vi "ThemalImaging(VDAQ)2.vi"() -> ()   [LabVIEW 2011]
uses:
  <vilib>/vision/Image Controls.llb/IMAQ Image.ctl
  <vilib>/Analysis/1siggen.llb/Riffle Array (I32).vi
  <vilib>/Analysis/NI_AALBase.lvlib
  <vilib>/vision/NI_Vision_Development_Module.lvlib
panel:
  out "数值":i32
  out "OnlineMap Array":T1[](array[typedef])
  out "Hue":i32
  out "Saturation":i32
  out "DR/R array":T1[](array[typedef])
  out "停止循环":bool
  out "imaging通知器输出":refnum<notifier>
  out "DeInitDSPs":i32
  out "错误输出":errorcluster
  in  "Stimuli":i32=5
  in  "FrameHeight":i32=576
  in  "FrameWidth":i32=704
  in  "选项卡控件":enum32{"前面板", "参数设置", "OnLineMap", "mask"}(tab)
  out "log":string
  out "Image":T1(plugin-control)
  out "Stim_ID":i32(listbox)=1
  in  "开始/暂停":bool=TRUE
  in  "停止":bool
  out "重排的 Stim ID":i32[](array[numeric]) caption="重排的{X}"
  out "重排的 Stim ID Index":i32[](array[numeric]) caption="重排的索引"
  in  "Contrast":i32(slide) min=0 max=127 scale=0.0..127.0
  in  "Brightness":i32(slide) min=0 max=255 scale=0.0..255.0
  in  "上限温度":dbl=32.5
  in  "下限温度":dbl=20.6
  out "当前点温度":dbl
  out "Histogram Graph":T2(graph) caption="直方图"
  out "校正循环计时":dbl caption="已用时间(s)"
  out "校准":bool
  out "start calibrate":bool
  out "wait calibrate":bool
  out "block":i32
  in  "FramesPerStim(25Hz)":i32=100
  in  "Blk目录":path=path "D:/_expt/111110_C27/Run_02_G4_ThemalImaging"
  in  "文件名":string="G4_E05"
  in  "TimeForPrepare(ms)":u32=1000
  in  "stim ID":u8[](array[numeric])=[0, 2, 4, 6, 8]
  in  "blk总数":i32=500
  in  "stim protocol":T3(array[ring])=[enum."prep stim", enum."wait calibrate", enum."wait respirator", enum."show stim", enum."recording data", enum."Blank stim", enum."write data", enum."DR/R", enum."ISI"]
  in  "blank stim":u8
  in  "wait（ms）":u32=10
  in  "ISI（ms）":u32=8000
  in  "stim 循环时间/秒":dbl=10.0
  in  "OnlineMap":cluster{"数组 1":i32[], "数组 2":i32[]}[](array[cluster])=[{"数组 1"=[2], "数组 2"=[6]}, {"数组 1"=[4], "数组 2"=[8]}, {"数组 1"=[2, 6], "数组 2"=[4, 8]}, {"数组 1"=[2, 4, 6, 8], "数组 2"=[0]}, {"数组 1"=[2, 4], "数组 2"=[6, 8]}]
  in  "DR/R parameter":T4={"frame_zero_0"=0, "frame_zero_1"=10, "frame_0"=40, "frame_1"=80}
  in  "mask 1":T1(plugin-control)=refnum
  in  "mask 2":T1(plugin-control)=refnum
  # "运行60秒后再开始"
  # "÷"
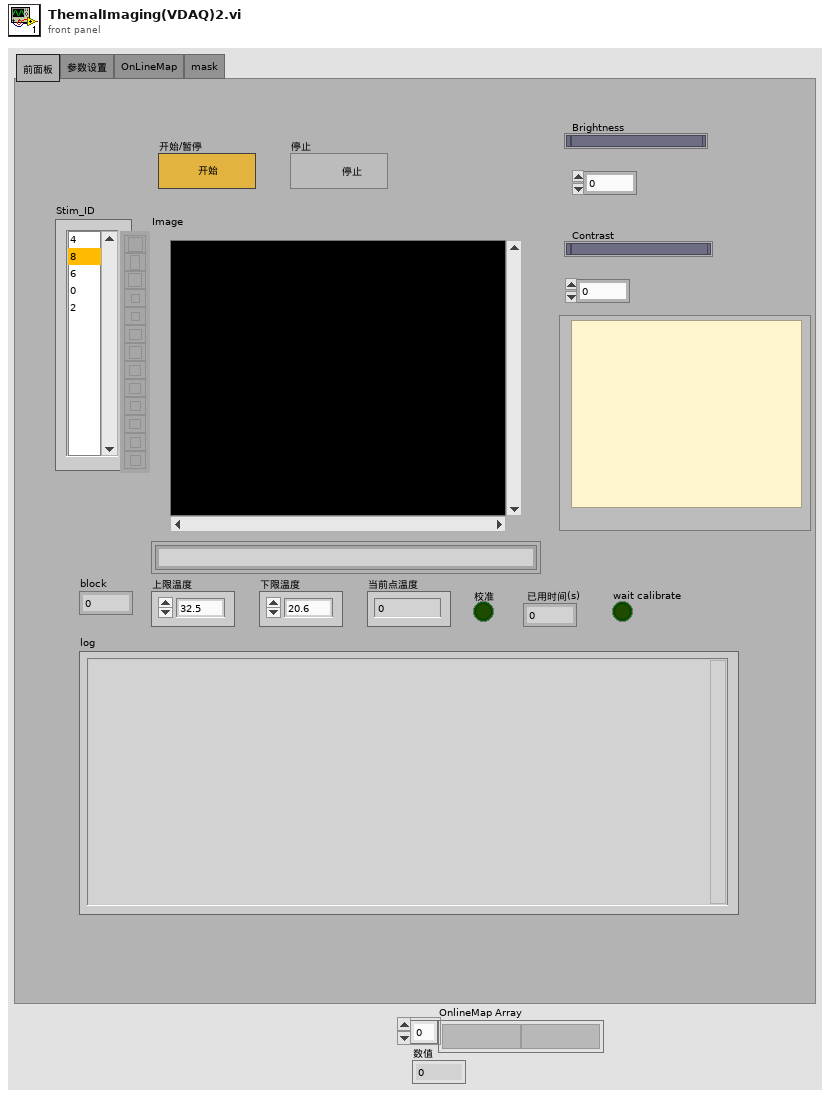
[diagram p1: front panel]
types:
  T1 = typedef "IMAQ Image.ctl" = refnum<image>
  T2 = cluster{"X Values":dbl[], "Histogram: h(x)":i32[]}
  T3 = enum16{"wait", "prep stim", "show stim", "wait respirator", "recording data", "write data", "Blank stim", "wait heart", "ISI", "DR/R", "wait calibrate"}[]
  T4 = cluster{"frame_zero_0":i32, "frame_zero_1":i32, "frame_0":i32, "frame_1":i32}
  T5 = typedef "Image Type" = u32
  T6 = enum16{"big-endian, network order", "native, host order", "little-endian"}
  T7 = cluster{"Mean Value":sgl, "Standard Variation":sgl, "Minimal Value":sgl, "Maximal Value":sgl, "Area (calibrated)":sgl, "Area (pixels)":u32, "%":sgl, "Calibration Valid":bool}
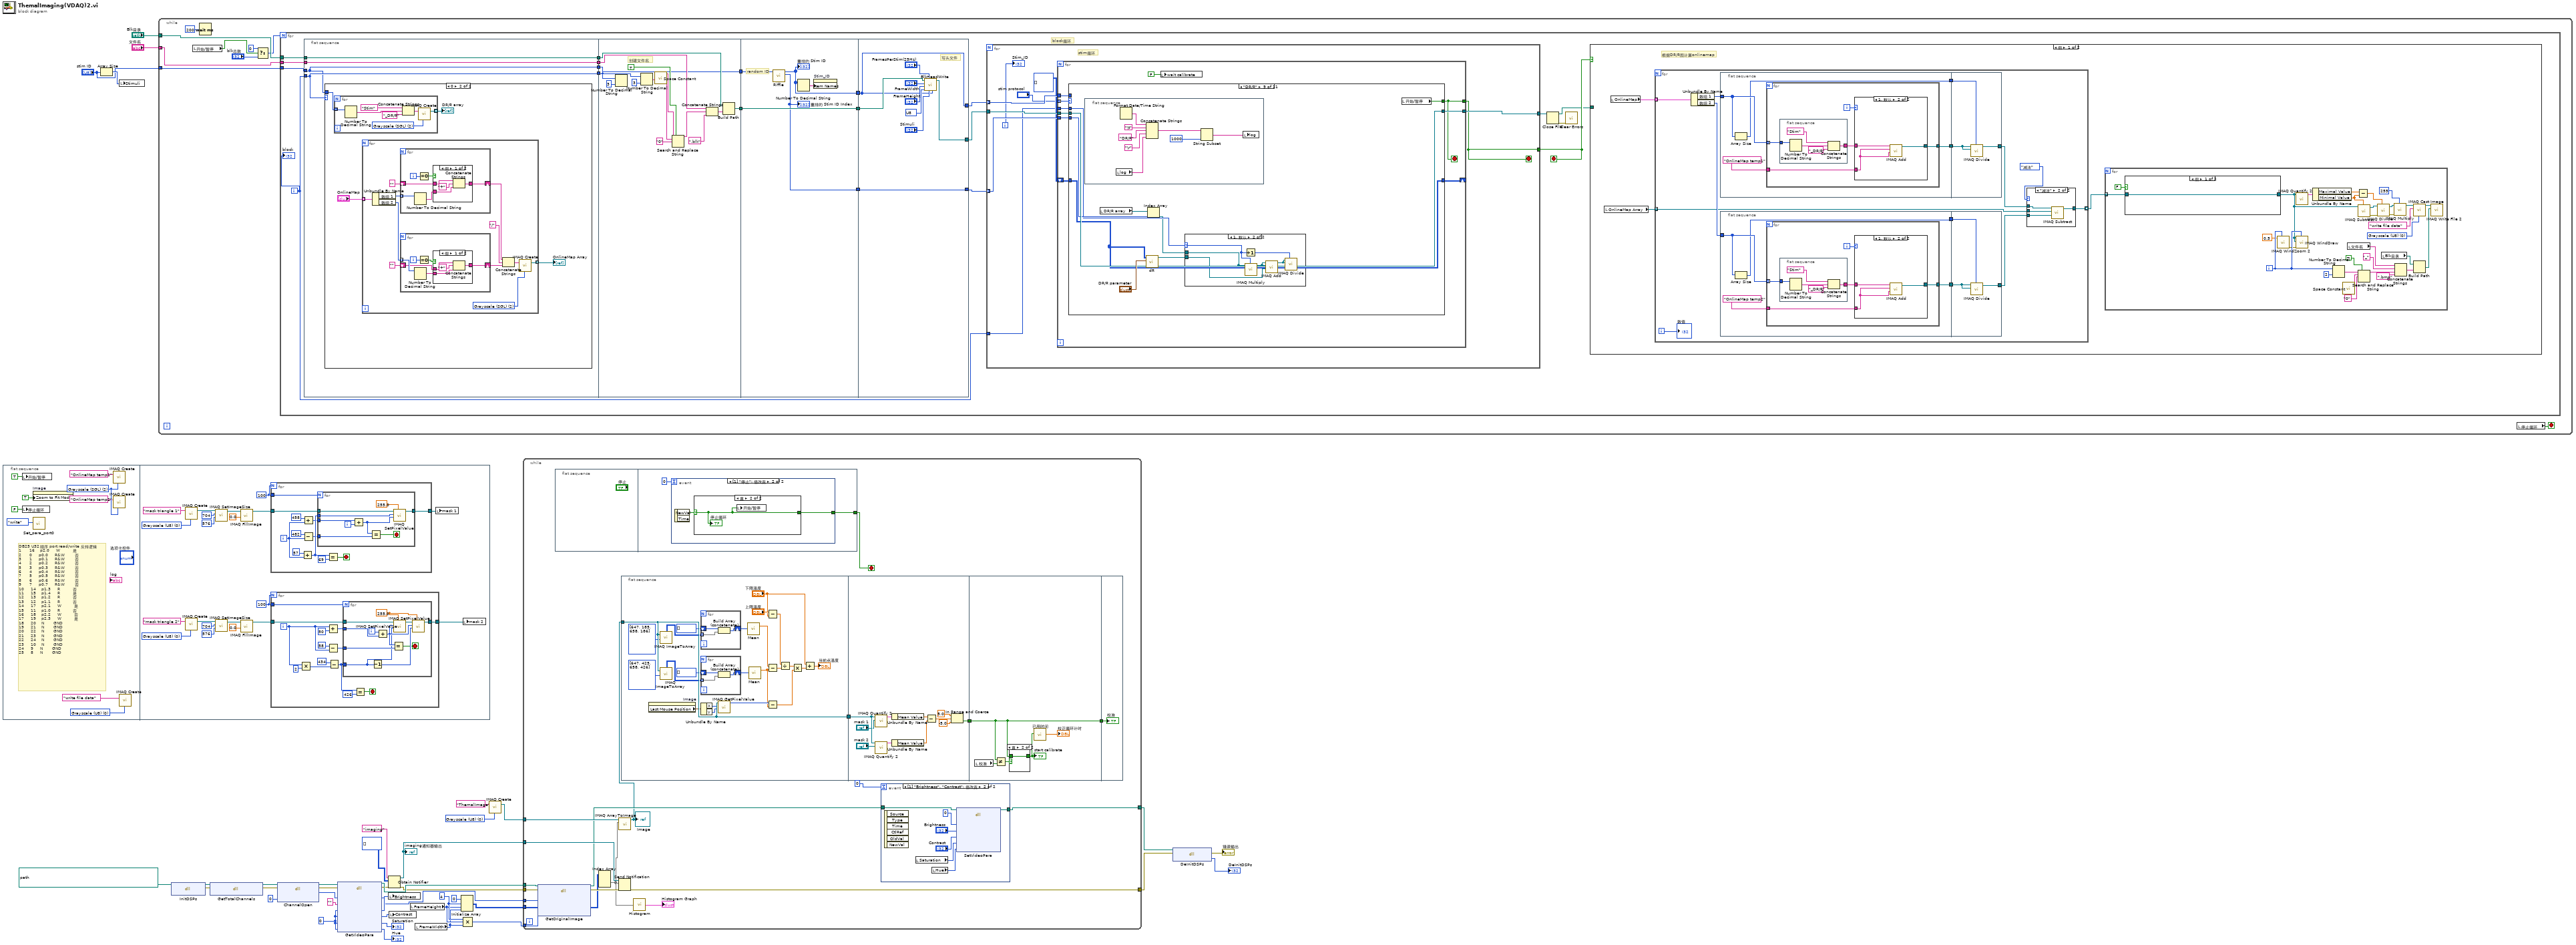
[diagram p0: block diagram]
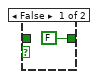
[diagram p2: hidden frame]
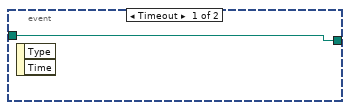
[diagram p3: hidden frame]
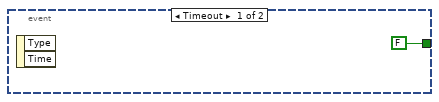
[diagram p4: hidden frame]
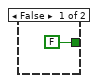
[diagram p5: hidden frame]
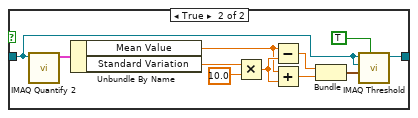
[diagram p6: hidden frame]
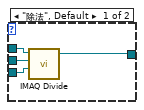
[diagram p7: hidden frame]
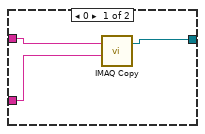
[diagram p8: hidden frame]
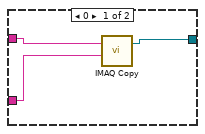
[diagram p9: hidden frame]
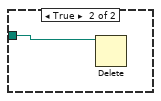
[diagram p10: hidden frame]
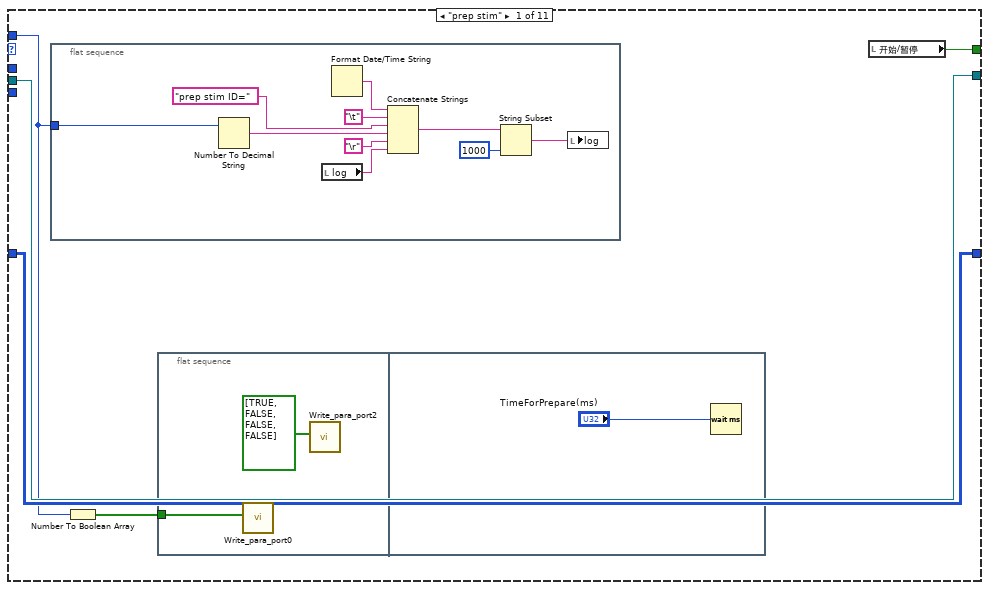
[diagram p14: hidden frame]
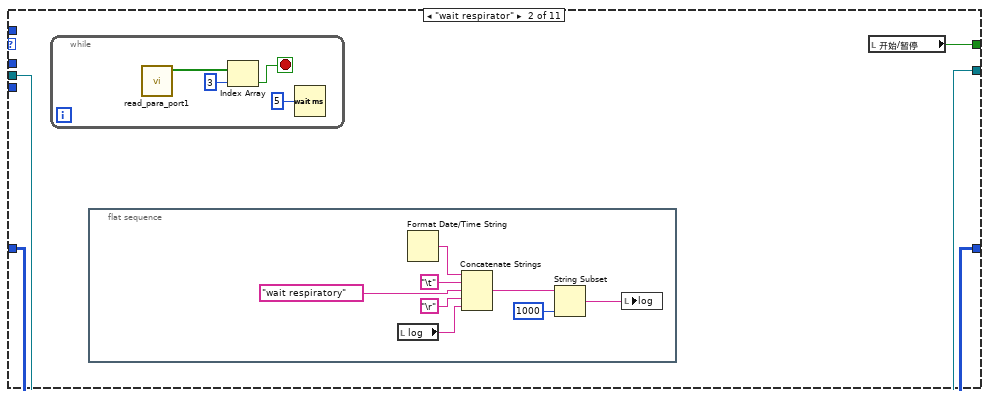
[diagram p15: hidden frame]
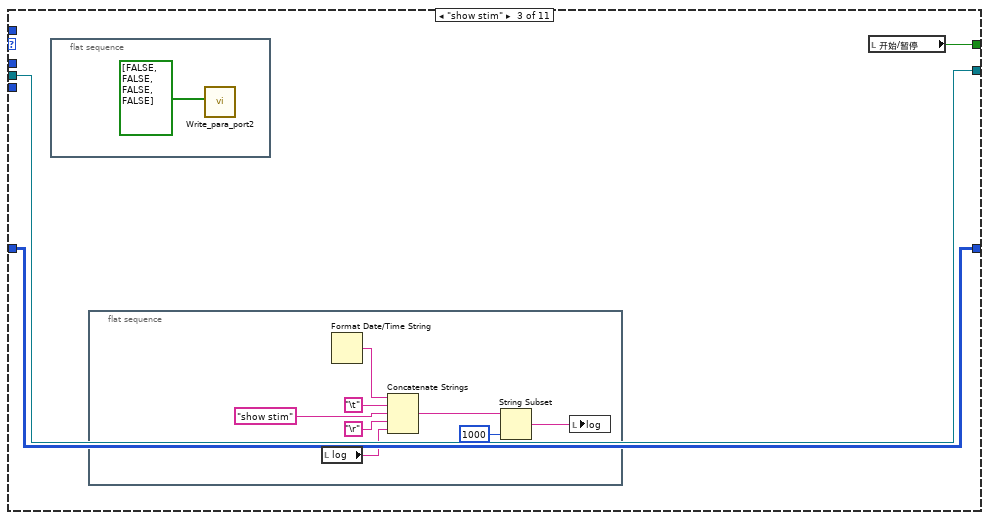
[diagram p16: hidden frame]
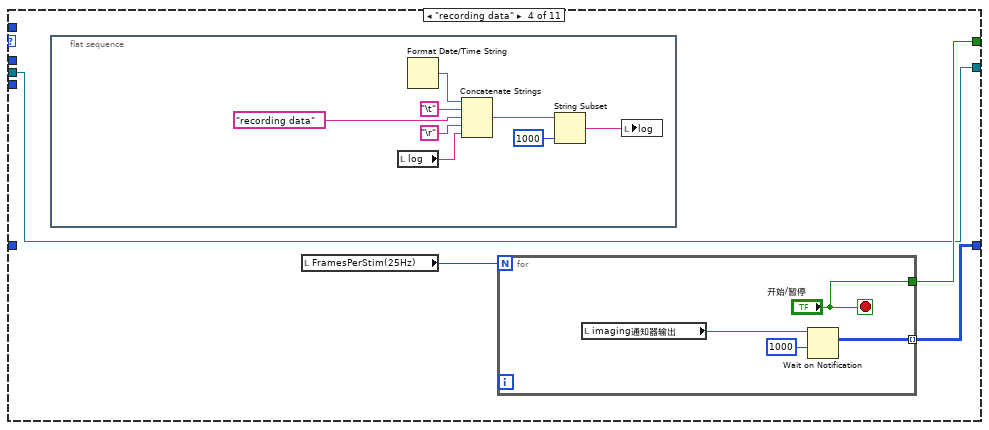
[diagram p17: hidden frame]
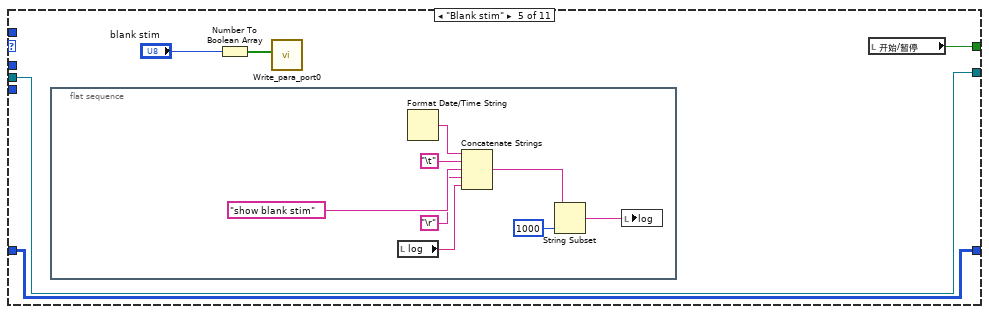
[diagram p18: hidden frame]
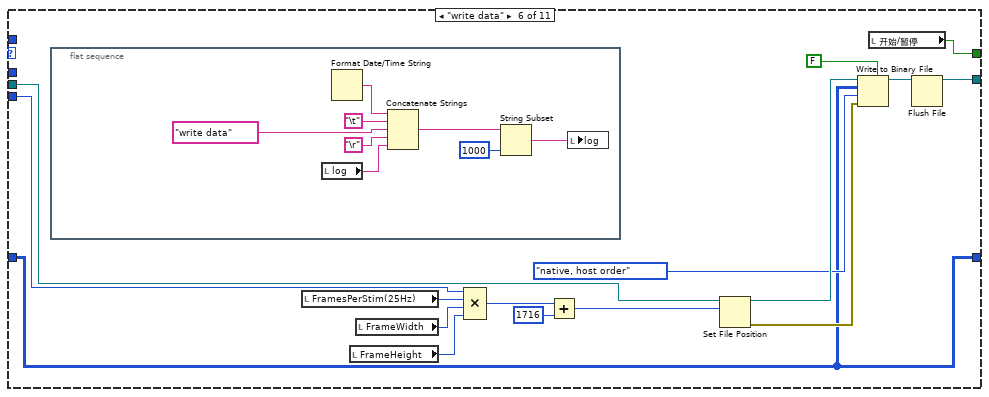
[diagram p19: hidden frame]
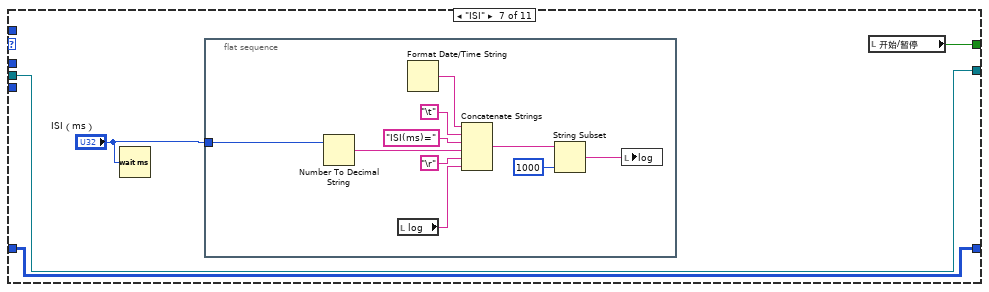
[diagram p20: hidden frame]
diagram:
  w17 = 4 ("元素")
  w34 = T5 0 items=["Grayscale (U8)", "Grayscale (I16)", "Grayscale (SGL)", "Complex (CSG)", "RGB (U32)", "HSL (U32)", "RGB (U64)", "Grayscale (U16)"] ("Image Type")
  w23 = 0 ("Brightness")
  n1 = flat-sequence {
    frame #0 {
      w40 = T5 0 items=["Grayscale (U8)", "Grayscale (I16)", "Grayscale (SGL)", "Complex (CSG)", "RGB (U32)", "HSL (U32)", "RGB (U64)", "Grayscale (U16)"] ("Image Type")
      w43 = T5 2 items=["Grayscale (U8)", "Grayscale (I16)", "Grayscale (SGL)", "Complex (CSG)", "RGB (U32)", "HSL (U32)", "RGB (U64)", "Grayscale (U16)"] ("Image Type")
      # "DB25\tU32顺序\tport\tread/write\t反转逻辑\n1\t     16\t   p2.0    \tW\t        是\n2\t     0    \tp0.0\t   \tR&W\t      否\n3\t     1\t\t   p0.1\t   \tR&W      \t否\n4\t\t    2\t   \tp0.2   \t\tR&W      \t否\n5\t\t    3\t\t   p0.3   \t\tR&W\t      否\n6\t\t    4\t   \tp0.4   \t\tR&W      \t否\n7\t\t    5\t   \tp0.5   \t\tR&W      \t否\n8\t\t    6\t   \tp0.6\t   \tR&W      \t否\n9\t    \t7\t   \tp0.7\t   \tR&W\t      否\n10\t    14   \tp1.3   \t\tR        \t否\n11\t   \t15   \tp1.4   \t\tR        \t是\n12\t   \t13   \tp1.2\t   \tR        \t否\n13    \t12   \tp1.1\t   \tR        \t否\n14     17   \tp2.1\t   \tW        \t是\n15    \t11   \tp1.0   \t\tR\t        否\n16    \t18   \tp2.2   \t\tW        \t否\n17    \t19\t   p2.3   \t\tW\t        是\n18    \t20   \tN   \t  \tGND\t\n19    \t21   \tN   \t  \tGND\t\n20\t    22\t   N\t  \t  \tGND\t\n21\t    23\t   N  \t  \t\tGND\t\n22\t    24\t   N  \t  \t\tGND\t\n23    \t10   \tN  \t  \t\tGND\t\n24    \t9\t    N  \t  \t\tGND\t\n25\t    8    \tN  \t  \t\tGND"
      n2 = local write "开始/暂停"(TRUE ("开始/暂停")) -> ()
      n3 = local write "停止循环"(FALSE ("开始/暂停")) -> ()
      n4 = property on="Image" class="ImageControl"("Zoom to Fit Mode"=TRUE) -> ()  [unwired: 2 in, 2 out]
      n5 = call "Set_para_port0.vi"("R or W"=enum16{"read", "write"}."write") -> ()  [unwired: 9 in, 2 out]
      n6 = call "IMAQ Create"("Image Name"="OnlineMap temp1", "Image Type"=w43) -> ()  [unwired: 3 in, 2 out]
      n7 = call "IMAQ Create"("Image Name"="OnlineMap temp2", "Image Type"=w43) -> ()  [unwired: 3 in, 2 out]
      n8 = call "IMAQ Create"("Image Name"="write file data", "Image Type"=w40) -> ()  [unwired: 3 in, 2 out]
    }
    frame #1 {
      w50 = 100
      w57 = T5 0 items=["Grayscale (U8)", "Grayscale (I16)", "Grayscale (SGL)", "Complex (CSG)", "RGB (U32)", "HSL (U32)", "RGB (U64)", "Grayscale (U16)"] ("Image Type")
      w60 = 100
      w67 = T5 0 items=["Grayscale (U8)", "Grayscale (I16)", "Grayscale (SGL)", "Complex (CSG)", "RGB (U32)", "HSL (U32)", "RGB (U64)", "Grayscale (U16)"] ("Image Type")
      n9 = call "IMAQ Create"("Image Name"="mask triangle 1", "Image Type"=w67) -> ("New Image"=w66:T1)  [unwired: 3 in, 1 out]
      n10 = call "IMAQ Create"("Image Name"="mask triangle 2", "Image Type"=w57) -> ("New Image"=w56:T1)  [unwired: 3 in, 1 out]
      n11 = call "IMAQ SetImageSize"("Y Resolution"=576, "X Resolution"=704, "Image"=w66) -> ("Image Out"=w63:T1)  [unwired: 2 in, 1 out]
      n12 = call "IMAQ SetImageSize"("Y Resolution"=576, "X Resolution"=704, "Image"=w56) -> ("Image Out"=w53:T1)  [unwired: 2 in, 1 out]
      n13 = call "IMAQ FillImage"("Pixel Value (U8, U16, I16, Float)"=sgl 0.0, "Image"=w63) -> ("Image Out"=w61:T1)  [unwired: 8 in, 1 out]
      n14 = call "IMAQ FillImage"("Pixel Value (U8, U16, I16, Float)"=sgl 0.0, "Image"=w53) -> ("Image Out"=w51:T1)  [unwired: 8 in, 1 out]
      n15 = for {
        N: w60 -> [_]
        tunnel: w60 -> [w105]
        tunnel: [w104] -> w59
        tunnel: w61 -> [w103]
        i -> [w95]
        stop <- w99 stop-if-true
        n16 = Add(x=57 ("X Coordinate"), y=w95) -> (x+y=w101:i32)
        n17 = Add(x=458 ("Y Coordinate"), y=w95) -> (x+y=w97:i32)
        n18 = Subtract(x=482 ("y"), y=w95) -> (x-y=w94:i32)
        n19 = for {
          N: w105 -> [_]
          tunnel: w103 -> [w114]
          tunnel: [w112] -> w104
          tunnel: w101 -> [w108]
          tunnel: w97 -> [w107]
          tunnel: w94 -> [w106]
          i -> [w111]
          stop <- w109 stop-if-true
          n20 = Add(x=w107, y=w111) -> (x+y=w110:i32)
          n21 = Equal?(x=w110, y=w106) -> (x = y?=w109:bool)
          n22 = call "IMAQ SetPixelValue"("Pixel Value"=sgl 255.0, "Y Coordinate"=w110, "X Coordinate"=w108, "Image"=w114) -> ("Image Out"=w112:T1)  [unwired: 6 in, 1 out]
        }
        n23 = Equal?(x=w101, y=69) -> (x = y?=w99:bool)
      }
      n24 = for {
        N: w50 -> [_]
        tunnel: w50 -> [w82]
        tunnel: [w81] -> w49
        tunnel: w51 -> [w80]
        i -> [w74]
        stop <- w69 stop-if-true
        n25 = Multiply(x=w74, y=2) -> (x*y=w72:i32)
        n26 = Add(x=w74, y=50 ("X Coordinate")) -> (x+y=w78:i32)
        n27 = Subtract(x=58 ("y"), y=w74) -> (x-y=w76:i32)
        n28 = Subtract(x=434 ("Y Coordinate"), y=w72) -> (x-y=w71:i32)
        n29 = for {
          N: w82 -> [_]
          tunnel: w80 -> [w93]
          tunnel: [w90] -> w81
          tunnel: w78 -> [w86]
          tunnel: w76 -> [w85]
          tunnel: w71 -> [w84]
          i -> [w92]
          stop <- w87 stop-if-true
          w83 = sgl 255.0 ("Pixel Value")
          n30 = Decrement(x=w84) -> (x-1=w89:i32)
          n31 = Add(x=w92, y=w86) -> (x+y=w88:i32)
          n32 = Equal?(x=w88, y=w85) -> (x = y?=w87:bool)
          n33 = call "IMAQ SetPixelValue"("Pixel Value"=w83, "Y Coordinate"=w84, "X Coordinate"=w88, "Image"=w93) -> ("Image Out"=w91:T1)  [unwired: 6 in, 1 out]
          n34 = call "IMAQ SetPixelValue"("Pixel Value"=w83, "Y Coordinate"=w89, "X Coordinate"=w88, "Image"=w91) -> ("Image Out"=w90:T1)  [unwired: 6 in, 1 out]
        }
        n35 = Equal?(x=w71, y=426) -> (x = y?=w69:bool)
      }
      n36 = local write "mask 1"(w59) -> ()
      n37 = local write "mask 2"(w49) -> ()
    }
  }
  n38 = Array Size(array="stim ID") -> (size(s)=w37:i32)
  n39 = local write "Stimuli"(w37) -> ()
  n40 = while {
    tunnel: "stim ID" -> [w123]
    tunnel: "文件名" -> [w122]
    tunnel: "Blk目录" -> [w121]
    stop <- w119 stop-if-true
    n41 = local read "开始/暂停"() -> (w118:bool)
    n42 = Wait (ms)(milliseconds to wait=u32 200 ("等待时间（毫秒）")) -> ()  [unwired: 1 out]
    n43 = Select(t=0, s=w118, f="blk总数") -> (s? t:f=w115:i32)
    n44 = for {
      N: w115 -> [_]
      tunnel: w123 -> [w128]
      tunnel: w122 -> [w143]
      tunnel: w121 -> [w142]
      i -> [w132]
      stop <- w134 stop-if-true
      # "block循环"
      n45 = flat-sequence {
        tunnel: w142 -> [w260]
        tunnel: w143 -> [w261]
        tunnel: w132 -> [w259]
        tunnel: [w259] -> w131
        tunnel: [w261] -> w130
        tunnel: [w260] -> w129
        tunnel: w128 -> [w258]
        tunnel: [w258] -> w126
        tunnel: [w307] -> w140
        tunnel: w131 -> [w313]
        tunnel: w130 -> [w312]
        tunnel: w129 -> [w308]
        tunnel: [w306] -> w127
        tunnel: w126 -> [w306]
        tunnel: w140 -> [w324]
        tunnel: [w324] -> w139
        tunnel: [w322] -> w138
        tunnel: w127 -> [w321]
        tunnel: [w320] -> w125
        tunnel: w139 -> [w328]
        tunnel: [w327] -> w141
        tunnel: w138 -> [w326]
        tunnel: [w326] -> w137
        tunnel: w125 -> [w325]
        tunnel: [w325] -> w124
        frame #0 {
          n46 = case shown="0" w259 {
            tunnel: w258 -> [_ w265]
            frame 1, Default {
            }
            frame 0 {
              n47 = for {
                tunnel: w265 -> [w302] mode=indexing
                tunnel: [w299] -> w264 mode=indexing
                w305 = T5 2 items=["Grayscale (U8)", "Grayscale (I16)", "Grayscale (SGL)", "Complex (CSG)", "RGB (U32)", "HSL (U32)", "RGB (U64)", "Grayscale (U16)"] ("Image Type")
                n48 = Number To Decimal String(number=w302) -> (decimal integer string=w303:string)  [unwired: 1 in]
                n49 = Concatenate Strings("Stim", w303, "_DR/R" ("字符串")) -> (w300:string)
                n50 = call "IMAQ Create"("Image Name"=w300, "Image Type"=w305) -> ("New Image"=w299:T1)  [unwired: 3 in, 1 out]
              }
              "DR/R array" <- w264
              n51 = for {
                tunnel: "OnlineMap" -> [w276] mode=indexing
                tunnel: [w266] -> w262 mode=indexing
                w274 = T5 2 items=["Grayscale (U8)", "Grayscale (I16)", "Grayscale (SGL)", "Complex (CSG)", "RGB (U32)", "HSL (U32)", "RGB (U64)", "Grayscale (U16)"] ("Image Type")
                n52 = Unbundle By Name(w276) -> ("数组 1"=w275:i32[], "数组 2"=w271:i32[])
                n53 = for {
                  tunnel: w275 -> [w291] mode=indexing
                  shift-right: [w289] -> w272
                  shift-left: "" -> [w288]
                  i -> [w293]
                  n54 = Number To Decimal String(number=w291) -> (decimal integer string=w290:string)  [unwired: 1 in]
                  n55 = Equal To 0?(x=w293) -> (x = 0?=w292:bool)
                  n56 = case shown="假" w292 {
                    tunnel: w290 -> [w294 w298]
                    tunnel: [w297 w298] -> w289
                    tunnel: w288 -> [w296 _]
                    frame False {
                      n57 = Concatenate Strings(w296, "+" ("字符串"), w294) -> (w297:string)
                    }
                    frame True {
                    }
                  }
                }
                n58 = for {
                  tunnel: w271 -> [w280] mode=indexing
                  shift-right: [w278] -> w269
                  shift-left: "" -> [w277]
                  i -> [w282]
                  n59 = Number To Decimal String(number=w280) -> (decimal integer string=w279:string)  [unwired: 1 in]
                  n60 = Equal To 0?(x=w282) -> (x = 0?=w281:bool)
                  n61 = case shown="假" w281 {
                    tunnel: w279 -> [w283 w287]
                    tunnel: [w286 w287] -> w278
                    tunnel: w277 -> [w285 _]
                    frame False {
                      n62 = Concatenate Strings(w285, "+" ("字符串"), w283) -> (w286:string)
                    }
                    frame True {
                    }
                  }
                }
                n63 = Concatenate Strings(w272, "/" ("字符串"), w269) -> (w267:string)
                n64 = call "IMAQ Create"("Image Name"=w267, "Image Type"=w274) -> ("New Image"=w266:T1)  [unwired: 3 in, 1 out]
              }
              "OnlineMap Array" <- w262
            }
          }
        }
        frame #1 {
          # "创建文件名"
          n65 = Number To Decimal String(number=w313, width (-)=i16 3 ("宽度(-)")) -> ()  [unwired: 1 out]
          n66 = Number To Decimal String(number=w313, width (-)=i16 3 ("宽度(-)")) -> (decimal integer string=w315:string)
          n67 = call <vilib>:"Space Constant.vi"() -> ("String"=w316:string)
          n68 = Search and Replace String(replace all?=TRUE ("替换全部？(F)"), input string=w315, search string=w316, replace string="0" ("替换字符串(\"\")")) -> (result string=w311:string)  [unwired: 4 in, 3 out]
          n69 = Concatenate Strings(w312, w311, ".blk" ("字符串")) -> (w309:string)
          n70 = Build Path(base path=w308, name or relative path=w309) -> (appended path=w307:path)
        }
        frame #2 {
          # "random ID"
          n71 = call-poly <vilib>:"Riffle.vi"("X"=w321) -> ("Riffled Index"=w320:i32[], "Riffled {X}"=w322:i32[])  [unwired: 8 in, 1 out]
          "重排的 Stim ID Index" <- w320
          "重排的 Stim ID" <- w322
          n72 = Number To Decimal String(number=w322) -> (decimal integer string=w323:string[])  [unwired: 1 in]
          n73 = property on="Stim_ID" class="LstBox (严格)"("Item Names"=w323) -> ()  [unwired: 2 in, 2 out]
        }
        frame #3 {
          w331 = u16 11 items=["U8"=11, "I16"=12, "U32"=13, "SGL"=14] ("datatype")
          # "写头文件"
          n74 = call "BlkHeadWrite.vi"("SequenceOfID"=w326, "Stimuli"="Stimuli", "FramesPerStim"="FramesPerStim(25Hz)", "datatype"=w331, "FrameHeight"="FrameHeight", "FrameWidth"="FrameWidth", "BlkFilePath"=w328) -> ("引用句柄输出"=w327:refnum<file>)  [unwired: 4 in]
        }
      }
      n75 = for {
        tunnel: w141 -> [w342]
        tunnel: [w340] -> w135
        tunnel: w124 -> [w341] mode=indexing
        tunnel: w137 -> [w339] mode=indexing
        tunnel: [w338] -> w134
        tunnel: w132 -> [w334]
        i -> [w337]
        stop <- w338 stop-if-true
        # "stim循环"
        n76 = for {
          tunnel: w341 -> [w351]
          tunnel: w339 -> [w349]
          tunnel: [w345] -> w338
          shift-right: [w348] -> _
          shift-left: u8[][][] [] ("初始化的数组") -> [w347]
          tunnel: "stim protocol" -> [w346] mode=indexing
          tunnel: w342 -> [w352]
          tunnel: [w350] -> w340
          tunnel: w334 -> [w344]
          stop <- w345 stop-if-true
          n77 = case shown="\"DR/R\"" w346 {
            tunnel: w352 -> [w354 w371 w386 w398 w414 w442 w452 w466 w486 w504 w522]
            tunnel: w351 -> [_ _ _ _ _ w441 _ _ w484 _ _]
            tunnel: [w354 w371 w386 w398 w414 w429 w452 w466 w486 w504 w522] -> w350
            tunnel: w349 -> [w353 _ _ _ _ _ _ _ _ _ _]
            tunnel: [w355 w372 w387 w400 w415 w427 w453 w467 w485 w505 w515] -> w345
            tunnel: [w356 w373 w388 w399 w416 w428 w454 w468 w479 w506 w521] -> w348
            tunnel: w347 -> [w356 w373 w388 _ w416 w428 w454 w468 w479 w506 w521]
            tunnel: w344 -> [_ _ _ _ _ _ _ _ w483 _ _]
            frame "prep stim" {
              n78 = flat-sequence {
                tunnel: w353 -> [w365]
                frame #0 {
                  n79 = Number To Decimal String(number=w365) -> (decimal integer string=w364:string)  [unwired: 1 in]
                  n80 = local read "log"() -> (w360:string)
                  n81 = Format Date/Time String() -> (date/time string=w367:string)  [unwired: 3 in]
                  n82 = Concatenate Strings(w367, "\t", "prep stim ID=" ("字符串"), w364, "\r", w360) -> (w362:string)
                  n83 = String Subset(string=w362, length (rest)=1000 ("y")) -> (substring=w361:string)  [unwired: 1 in]
                  n84 = local write "log"(w361) -> ()
                }
              }
              n85 = Number To Boolean Array(number=w353) -> (Boolean array=w357:bool[])
              n86 = flat-sequence {
                tunnel: w357 -> [w369]
                frame #0 {
                  n87 = call "Write_para_port0.vi"("port0（8元素）"=w369) -> ()  [unwired: 10 in, 1 out]
                  n88 = call "Write_para_port2.vi"("port2（4元素）"=bool[] [TRUE, FALSE, FALSE, FALSE] ("port2")) -> ()  [unwired: 10 in, 1 out]
                }
                frame #1 {
                  n89 = Wait (ms)(milliseconds to wait="TimeForPrepare(ms)") -> ()  [unwired: 1 out]
                }
              }
              n90 = local read "开始/暂停"() -> (w355:bool)
            }
            frame "wait respirator" {
              n91 = while {
                stop <- w383 stop-if-true
                n92 = call "read_para_port1.vi"() -> ("port1（5元素）"=w385:bool[])  [unwired: 10 in, 1 out]
                n93 = Index Array(array=w385, index=3 ("索引")) -> (element=w383:bool)
                n94 = Wait (ms)(milliseconds to wait=u32 5 ("等待时间（毫秒）")) -> ()  [unwired: 1 out]
              }
              n95 = flat-sequence {
                frame #0 {
                  n96 = local read "log"() -> (w376:string)
                  n97 = Format Date/Time String() -> (date/time string=w381:string)  [unwired: 3 in]
                  n98 = Concatenate Strings(w381, "\t", "wait respiratory" ("字符串"), "\r", w376) -> (w378:string)
                  n99 = String Subset(string=w378, length (rest)=1000 ("y")) -> (substring=w377:string)  [unwired: 1 in]
                  n100 = local write "log"(w377) -> ()
                }
              }
              n101 = local read "开始/暂停"() -> (w372:bool)
            }
            frame "show stim" {
              n102 = flat-sequence {
                frame #0 {
                  n103 = call "Write_para_port2.vi"("port2（4元素）"=bool[] [FALSE, FALSE, FALSE, FALSE] ("port2")) -> ()  [unwired: 10 in, 1 out]
                }
              }
              n104 = flat-sequence {
                frame #0 {
                  n105 = local read "log"() -> (w391:string)
                  n106 = Format Date/Time String() -> (date/time string=w396:string)  [unwired: 3 in]
                  n107 = Concatenate Strings(w396, "\t", "show stim" ("字符串"), "\r", w391) -> (w393:string)
                  n108 = String Subset(string=w393, length (rest)=1000 ("y")) -> (substring=w392:string)  [unwired: 1 in]
                  n109 = local write "log"(w392) -> ()
                }
              }
              n110 = local read "开始/暂停"() -> (w387:bool)
            }
            frame "recording data" {
              n111 = flat-sequence {
                frame #0 {
                  n112 = local read "log"() -> (w404:string)
                  n113 = Format Date/Time String() -> (date/time string=w409:string)  [unwired: 3 in]
                  n114 = Concatenate Strings(w409, "\t", "recording data" ("字符串"), "\r", w404) -> (w406:string)
                  n115 = String Subset(string=w406, length (rest)=1000 ("y")) -> (substring=w405:string)  [unwired: 1 in]
                  n116 = local write "log"(w405) -> ()
                }
              }
              n117 = local read "FramesPerStim(25Hz)"() -> (w401:i32)
              n118 = for {
                N: w401 -> [_]
                tunnel: [w412] -> w399 mode=indexing
                tunnel: ["开始/暂停"] -> w400
                stop <- "开始/暂停" stop-if-true
                n119 = local read "imaging通知器输出"() -> (w413:refnum<notifier>)
                n120 = Wait on Notification(notifier=w413, timeout in ms (-1)=1000 ("超时毫秒(-1)")) -> (notification=w412:u8[][])  [unwired: 2 in, 3 out]
              }
            }
            frame "Blank stim" {
              n121 = flat-sequence {
                frame #0 {
                  n122 = local read "log"() -> (w421:string)
                  n123 = Format Date/Time String() -> (date/time string=w426:string)  [unwired: 3 in]
                  n124 = Concatenate Strings(w426, "\t", "show blank stim" ("字符串"), "\r", w421) -> (w423:string)
                  n125 = String Subset(string=w423, length (rest)=1000 ("y")) -> (substring=w422:string)  [unwired: 1 in]
                  n126 = local write "log"(w422) -> ()
                }
              }
              n127 = Number To Boolean Array(number="blank stim") -> (Boolean array=w417:bool[])
              n128 = call "Write_para_port0.vi"("port0（8元素）"=w417) -> ()  [unwired: 10 in, 1 out]
              n129 = local read "开始/暂停"() -> (w415:bool)
            }
            frame "write data" {
              n130 = flat-sequence {
                frame #0 {
                  n131 = local read "log"() -> (w445:string)
                  n132 = Format Date/Time String() -> (date/time string=w450:string)  [unwired: 3 in]
                  n133 = Concatenate Strings(w450, "\t", "write data" ("字符串"), "\r", w445) -> (w447:string)
                  n134 = String Subset(string=w447, length (rest)=1000 ("y")) -> (substring=w446:string)  [unwired: 1 in]
                  n135 = local write "log"(w446) -> ()
                }
              }
              n136 = local read "FramesPerStim(25Hz)"() -> (w433:i32)
              n137 = local read "FrameHeight"() -> (w431:i32)
              n138 = local read "FrameWidth"() -> (w432:i32)
              n139 = Compound Arithmetic op=MULTIPLY(w441, w433, w432, w431) -> (w436:i32)
              n140 = Add(x=w436, y=i64 1716 ("偏移量（字节）（0）")) -> (x+y=w434:i64)
              n141 = Set File Position(offset (in bytes) (0)=w434, refnum=w442) -> (refnum out=w439:refnum<file>, error out=w437:errorcluster)  [unwired: 2 in]
              n142 = Write to Binary File(file (use dialog)=w439, data=w428, error in=w437, 5:FALSE ("预置数组或字符串大小？(T)"), 9:T6."native, host order" ("字节顺序(0:big-endian, network order)")) -> (refnum out=w430:refnum<file>)  [unwired: 1 in, 2 out]
              n143 = local read "开始/暂停"() -> (w427:bool)
              n144 = Flush File(refnum=w430) -> (refnum out=w429:refnum<file>)  [unwired: 1 in, 1 out]
            }
            frame "ISI" {
              n145 = Wait (ms)(milliseconds to wait="ISI（ms）") -> ()  [unwired: 1 out]
              n146 = flat-sequence {
                tunnel: "ISI（ms）" -> [w458]
                frame #0 {
                  n147 = Number To Decimal String(number=w458) -> (decimal integer string=w462:string)  [unwired: 1 in]
                  n148 = local read "log"() -> (w457:string)
                  n149 = Format Date/Time String() -> (date/time string=w464:string)  [unwired: 3 in]
                  n150 = Concatenate Strings(w464, "\t", "ISI(ms)=" ("字符串"), w462, "\r", w457) -> (w460:string)
                  n151 = String Subset(string=w460, length (rest)=1000 ("y")) -> (substring=w459:string)  [unwired: 1 in]
                  n152 = local write "log"(w459) -> ()
                }
              }
              n153 = local read "开始/暂停"() -> (w453:bool)
            }
            frame "wait", Default {
              n154 = Wait (ms)(milliseconds to wait="wait（ms）") -> ()  [unwired: 1 out]
              n155 = flat-sequence {
                tunnel: "wait（ms）" -> [w472]
                frame #0 {
                  n156 = Number To Decimal String(number=w472) -> (decimal integer string=w476:string)  [unwired: 1 in]
                  n157 = local read "log"() -> (w471:string)
                  n158 = Format Date/Time String() -> (date/time string=w478:string)  [unwired: 3 in]
                  n159 = Concatenate Strings(w478, "\t", "wait(ms)=" ("字符串"), w476, "\r", w471) -> (w474:string)
                  n160 = String Subset(string=w474, length (rest)=1000 ("y")) -> (substring=w473:string)  [unwired: 1 in]
                  n161 = local write "log"(w473) -> ()
                }
              }
              n162 = local read "开始/暂停"() -> (w467:bool)
            }
            frame "DR/R" {
              n163 = flat-sequence {
                frame #0 {
                  n164 = local read "log"() -> (w490:string)
                  n165 = Format Date/Time String() -> (date/time string=w495:string)  [unwired: 3 in]
                  n166 = Concatenate Strings(w495, "\t", "DR/R" ("字符串"), "\r", w490) -> (w492:string)
                  n167 = String Subset(string=w492, length (rest)=1000 ("y")) -> (substring=w491:string)  [unwired: 1 in]
                  n168 = local write "log"(w491) -> ()
                }
              }
              n169 = local read "DR/R array"() -> (w480:T1[])
              n170 = call "dR.vi"("DR/R parameter"="DR/R parameter", "数组"=w479) -> ("Image Dst Out"=w482:T1)  [unwired: 9 in]
              n171 = Index Array(array=w480, index=w484) -> (element=w481:T1)
              n172 = case shown="1, 默认" w483 {
                selector: w483 -> [_ w500]
                tunnel: w482 -> [w497 w501]
                tunnel: w481 -> [w496 w503]
                frame 0 {
                  n173 = call "IMAQ Copy"("Image Dst"=w496, "Image Src"=w497) -> ()  [unwired: 4 in, 2 out]
                }
                frame 1, Default {
                  n174 = Increment(x=w500) -> (x+1=w499:i32)
                  n175 = call "IMAQ Multiply"("Image Src A"=w503, "Constant"=w500, "Image Dst"=w503) -> ("Image Dst Out"=w502:T1)  [unwired: 4 in, 1 out]
                  n176 = call "IMAQ Add"("Image Src A"=w502, "Image Dst"=w502, "Image Src B"=w501) -> ("Image Dst Out"=w498:T1)  [unwired: 4 in, 1 out]
                  n177 = call "IMAQ Divide"("Image Src A"=w498, "Constant"=w499, "Image Dst"=w498) -> ()  [unwired: 4 in, 2 out]
                }
              }
              n178 = local read "开始/暂停"() -> (w485:bool)
            }
            frame "wait heart" {
              n179 = flat-sequence {
                frame #0 {
                  n180 = local read "log"() -> (w509:string)
                  n181 = Format Date/Time String() -> (date/time string=w514:string)  [unwired: 3 in]
                  n182 = Concatenate Strings(w514, "\t", "wait heart" ("字符串"), "\r", w509) -> (w511:string)
                  n183 = String Subset(string=w511, length (rest)=1000 ("y")) -> (substring=w510:string)  [unwired: 1 in]
                  n184 = local write "log"(w510) -> ()
                }
              }
              n185 = local read "开始/暂停"() -> (w505:bool)
            }
            frame "wait calibrate" {
              n186 = local read "校正循环计时"() -> (w520:dbl)
              n187 = Subtract(x=60.0, y=w520) -> (x-y=w518:dbl)
              n188 = Less Or Equal?(x=w518, y="stim 循环时间/秒") -> (x <= y?=w516:bool)
              n189 = case shown="真" w516 {
                selector: w516 -> [_ w525]
                tunnel: [FALSE ("开始/暂停") w524] -> w515
                frame False {
                }
                frame True {
                  n190 = flat-sequence {
                    tunnel: [w526] -> w524
                    frame #0 {
                      n191 = while {
                        tunnel: [w527] -> w526
                        stop <- w528 stop-if-true
                        n192 = local read "start calibrate"() -> (w529:bool)
                        n193 = local read "开始/暂停"() -> (w527:bool)
                        n194 = Wait (ms)(milliseconds to wait=u32 5 ("等待时间（毫秒）")) -> ()  [unwired: 1 out]
                        n195 = Or(x=w529, y=w527) -> (x .or. y?=w528:bool)
                      }
                    }
                    frame #1 {
                      n196 = Wait (ms)(milliseconds to wait=u32 3000 ("等待时间（毫秒）")) -> ()  [unwired: 1 out]
                    }
                  }
                  "wait calibrate" <- w525
                }
              }
            }
          }
          n197 = local write "wait calibrate"(FALSE ("wait calibrate")) -> ()
        }
        "Stim_ID" <- w337
      }
      n198 = Close File(refnum=w135) -> (path=w133:path, error out=w136:errorcluster)  [unwired: 1 in]
      n199 = call <vilib>:"Clear Errors.vi"("error in (no error)"=w136) -> ()  [unwired: 6 in, 1 out]
      n200 = case shown="假" w134 {
        tunnel: w133 -> [_ w257]
        frame False {
          # "根据DR/R图计算onlinemap"
          n201 = local read "OnlineMap Array"() -> (w145:T1[])
          n202 = local read "OnlineMap"() -> (w146:cluster{"数组 1":i32[], "数组 2":i32[]}[])
          n203 = for {
            tunnel: w146 -> [w202] mode=indexing
            tunnel: w145 -> [w193] mode=indexing
            tunnel: [w191] -> w144 mode=indexing
            i -> [w190]
            n204 = Unbundle By Name(w202) -> ("数组 1"=w201:i32[], "数组 2"=w196:i32[])
            n205 = flat-sequence {
              tunnel: w201 -> [w236]
              tunnel: [w235] -> w200
              tunnel: [w234] -> w199
              tunnel: w200 -> [w255]
              tunnel: w199 -> [w256]
              tunnel: [w254] -> w195
              frame #0 {
                n206 = Array Size(array=w236) -> (size(s)=w234:i32)
                n207 = for {
                  tunnel: w236 -> [w242] mode=indexing
                  tunnel: "OnlineMap temp1" ("Image Name") -> [w240]
                  tunnel: [w238] -> w235
                  i -> [w239]
                  n208 = flat-sequence {
                    tunnel: w242 -> [w251]
                    tunnel: [w249] -> w241
                    frame #0 {
                      n209 = Number To Decimal String(number=w251) -> (decimal integer string=w252:string)  [unwired: 1 in]
                      n210 = Concatenate Strings("Stim", w252, "_DR/R" ("字符串")) -> (w249:string)
                    }
                  }
                  n211 = case shown="1, 默认" w239 {
                    tunnel: w241 -> [w245 w248]
                    tunnel: w240 -> [w244 w247]
                    tunnel: [w243 w246] -> w238
                    frame 0 {
                      n212 = call "IMAQ Copy"("Image Dst"=w244, "Image Src"=w245) -> ("Image Dst Out"=w243:T1)  [unwired: 4 in, 1 out]
                    }
                    frame 1, Default {
                      n213 = call "IMAQ Add"("Image Src A"=w248, "Image Dst"=w247, "Image Src B"=w247) -> ("Image Dst Out"=w246:T1)  [unwired: 4 in, 1 out]
                    }
                  }
                }
              }
              frame #1 {
                n214 = call "IMAQ Divide"("Image Src A"=w255, "Constant"=w256, "Image Dst"=w255) -> ("Image Dst Out"=w254:T1)  [unwired: 4 in, 1 out]
              }
            }
            n215 = flat-sequence {
              tunnel: w196 -> [w213]
              tunnel: [w212] -> w198
              tunnel: [w211] -> w197
              tunnel: w198 -> [w232]
              tunnel: w197 -> [w233]
              tunnel: [w231] -> w194
              frame #0 {
                n216 = Array Size(array=w213) -> (size(s)=w211:i32)
                n217 = for {
                  tunnel: w213 -> [w219] mode=indexing
                  tunnel: "OnlineMap temp2" ("Image Name") -> [w217]
                  tunnel: [w215] -> w212
                  i -> [w216]
                  n218 = flat-sequence {
                    tunnel: w219 -> [w228]
                    tunnel: [w226] -> w218
                    frame #0 {
                      n219 = Number To Decimal String(number=w228) -> (decimal integer string=w229:string)  [unwired: 1 in]
                      n220 = Concatenate Strings("Stim", w229, "_DR/R" ("字符串")) -> (w226:string)
                    }
                  }
                  n221 = case shown="1, 默认" w216 {
                    tunnel: w218 -> [w222 w225]
                    tunnel: w217 -> [w221 w224]
                    tunnel: [w220 w223] -> w215
                    frame 0 {
                      n222 = call "IMAQ Copy"("Image Dst"=w221, "Image Src"=w222) -> ("Image Dst Out"=w220:T1)  [unwired: 4 in, 1 out]
                    }
                    frame 1, Default {
                      n223 = call "IMAQ Add"("Image Src A"=w225, "Image Dst"=w224, "Image Src B"=w224) -> ("Image Dst Out"=w223:T1)  [unwired: 4 in, 1 out]
                    }
                  }
                }
              }
              frame #1 {
                n224 = call "IMAQ Divide"("Image Src A"=w232, "Constant"=w233, "Image Dst"=w232) -> ("Image Dst Out"=w231:T1)  [unwired: 4 in, 1 out]
              }
            }
            n225 = case shown="\"减法\"" enum16{"除法", "减法"}."减法" {
              tunnel: w195 -> [w206 w210]
              tunnel: w194 -> [w205 w209]
              tunnel: w193 -> [w204 w208]
              tunnel: [w203 w207] -> w191
              frame "除法", Default {
                n226 = call "IMAQ Divide"("Image Src A"=w206, "Image Dst"=w204, "Image Src B"=w205) -> ("Image Dst Out"=w203:T1)  [unwired: 4 in, 1 out]
              }
              frame "减法" {
                n227 = call "IMAQ Subtract"("Image Src A"=w210, "Image Dst"=w208, "Image Src B"=w209) -> ("Image Dst Out"=w207:T1)  [unwired: 4 in, 1 out]
              }
            }
            "数值" <- w190
          }
          n228 = for {
            tunnel: w144 -> [w177] mode=indexing
            i -> [w175]
            w161 = T5 0 items=["Grayscale (U8)", "Grayscale (I16)", "Grayscale (SGL)", "Complex (CSG)", "RGB (U32)", "HSL (U32)", "RGB (U64)", "Grayscale (U16)"] ("Image Type")
            n229 = case shown="假" FALSE {
              tunnel: [w178 w183] -> w156
              tunnel: w177 -> [w178 w182]
              frame False {
              }
              frame True {
                n230 = call "IMAQ Quantify 2"("Image"=w182) -> ("Global Report"=w189:T7)  [unwired: 8 in, 2 out]
                n231 = Unbundle By Name(w189) -> ("Mean Value"=w181:sgl, "Standard Variation"=w180:sgl)
                n232 = Multiply(x=w180, y=sgl 10.0) -> (x*y=w187:sgl)
                n233 = Subtract(x=w181, y=w187) -> (x-y=w186:sgl)
                n234 = Add(x=w181, y=w187) -> (x+y=w185:sgl)
                n235 = Bundle(w186, w185) -> (w184:cluster{sgl, sgl})  [unwired: 1 in]
                n236 = call "IMAQ Threshold"("Keep/Replace Value (Replace)"=TRUE, "Range"=w184, "Image Dst"=w182, "Image Src"=w182) -> ("Image Dst Out"=w183:T1)  [unwired: 6 in, 1 out]
              }
            }
            n237 = call "IMAQ WindZoom 2"("Window Number (0...15)"=w175, "Zoom Factor"=sgl 0.5) -> ("error out"=w157:errorcluster)  [unwired: 6 in, 3 out]
            n238 = call "IMAQ Quantify 2"("Image"=w156) -> ("Global Report"=w159:T7)  [unwired: 8 in, 2 out]
            n239 = call "IMAQ WindDraw"("Window Number (0...15)"=w175, "error in (no error)"=w157, "Title"=w156, "Image"=w156) -> ()  [unwired: 6 in, 2 out]
            n240 = Unbundle By Name(w159) -> ("Maximal Value"=w158:sgl, "Minimal Value"=w155:sgl)
            n241 = Number To Decimal String(number=w175, width (-)=i16 2 ("宽度(-)")) -> (decimal integer string=w171:string)
            n242 = call <vilib>:"Space Constant.vi"() -> ("String"=w170:string)
            n243 = local read "文件名"() -> (w173:string)
            n244 = Subtract(x=w158, y=w155) -> (x-y=w152:sgl)
            n245 = call "IMAQ Subtract"("Image Src A"=w156, "Constant"=w155) -> ("Image Dst Out"=w153:T1, "error out"=w154:errorcluster)  [unwired: 5 in]
            n246 = Search and Replace String(replace all?=TRUE ("替换全部？(F)"), input string=w171, search string=w170, replace string="0" ("替换字符串(\"\")")) -> (result string=w166:string)  [unwired: 4 in, 3 out]
            n247 = call "IMAQ Divide"("Image Src A"=w153, "Constant"=w152, "error in (no error)"=w154) -> ("Image Dst Out"=w150:T1, "error out"=w151:errorcluster)  [unwired: 4 in]
            n248 = local read "Blk目录"() -> (w164:path)
            n249 = call "IMAQ Multiply"("Image Src A"=w150, "Constant"=255, "error in (no error)"=w151) -> ("Image Dst Out"=w148:T1)  [unwired: 4 in, 1 out]
            n250 = Concatenate Strings(w173, "_" ("字符串"), w166, ".bmp" ("字符串")) -> (w163:string)
            n251 = call "IMAQ Cast Image"("Image Type"=w161, "Image Dst"="write file data" ("替换字符串(\"\")"), "Image Src"=w148) -> ("Image Dst Out"=w160:T1)  [unwired: 7 in, 1 out]
            n252 = Build Path(base path=w164, name or relative path=w163) -> (appended path=w162:path)
            n253 = call-poly "IMAQ Write File 2"("File Path"=w162, "Image"=w160) -> ()  [unwired: 8 in, 2 out]
          }
        }
        frame True {
          n254 = Delete(path (use dialog)=w257) -> ()  [unwired: 4 in, 3 out]
        }
      }
      "block" <- w132
    }
    n255 = local read "停止循环"() -> (w119:bool)
  }
  n256 = dll-call lib="PTH1labs C\nProgram Files\tHikvision+DS-4000系列板卡SDK and Demo Version 5.1SDKcard sdk\nDs40xxSDK.dll" fn="InitDSPs"(path in=path "C:/Program Files/Hikvision/DS-4000系列板卡SDK and Demo Version 5.1/SDK/card sdk/Ds40xxSDK.dll" ("路径输入")) -> (path out=w19:path, error out=w29:errorcluster)  [unwired: 2 in, 1 out]
  n257 = dll-call lib="PTH1labs C\nProgram Files\tHikvision+DS-4000系列板卡SDK and Demo Version 5.1SDKcard sdk\nDs40xxSDK.dll" fn="GetTotalChannels"(path in=w19, error in=w29) -> (path out=w21:path, error out=w30:errorcluster)  [unwired: 1 in, 1 out]
  n258 = dll-call lib="PTH1labs C\nProgram Files\tHikvision+DS-4000系列板卡SDK and Demo Version 5.1SDKcard sdk\nDs40xxSDK.dll" fn="ChannelOpen"(path in=w21, error in=w30, "ChannelNum"=0) -> (path out=w26:path, error out=w31:errorcluster, "返回类型"=w27:u32)  [unwired: 2 in]
  n259 = dll-call lib="PTH1babs C\nProgram Files\tHikvision+DS-4000系列板卡SDK and Demo Version 5.1Bin\nDs40xxSDK.dll" fn="GetVideoPara"(path in=w26, error in=w31, "hChannelHandle"=w27, "VideoStandard"="", "Brightness"=w23, "Contrast"=w23, "Saturation"=w23, "Hue"=w23) -> (path out=w13:path, error out=w9:errorcluster, "hChannelHandle"=w12:u32, "Brightness"=w25:i32, "Contrast"=w24:i32, "Saturation"=→"Saturation":i32, "Hue"=→"Hue":i32)  [unwired: 1 in, 2 out]
  n260 = Obtain Notifier(name (unnamed)="imaging" ("名称（未命名）"), notification data type=u8[][] [] ("初始化的数组"), error in (no error)=w9) -> (notifier out=w7:refnum<notifier>, error out=w8:errorcluster)  [unwired: 1 in, 1 out]
  "imaging通知器输出" <- w7
  n261 = local write "Brightness"(w25) -> ()
  n262 = local write "Contrast"(w24) -> ()
  n263 = local read "FrameHeight"() -> (w16:i32)
  n264 = local read "FrameWidth"() -> (w15:i32)
  n265 = Initialize Array(u8 0 ("元素"), w17, w16, w15) -> (w10:u8[][][])
  n266 = Compound Arithmetic op=MULTIPLY(w17, w16, w15) -> (w14:i32)
  n267 = call "IMAQ Create"("Image Name"="ThemalImage", "Image Type"=w34) -> ("New Image"=w3:T1)  [unwired: 2 in, 2 out]
  n268 = while {
    tunnel: w10 -> [w551]
    tunnel: w14 -> [w550]
    tunnel: w12 -> [w549]
    tunnel: w13 -> [w548]
    tunnel: w8 -> [w547]
    tunnel: w7 -> [w546]
    tunnel: [w543] -> w5
    tunnel: [w539] -> w4
    tunnel: w3 -> [w542]
    stop <- w541 stop-if-true
    n269 = dll-call lib="PTH1labs C\nProgram Files\tHikvision+DS-4000系列板卡SDK and Demo Version 5.1SDKcard sdk\nDs40xxSDK.dll" fn="GetOriginalImage"(path in=w548, error in=w547, "hChannelHandle"=w549, "ImageBuf"=w551, "Size"=w550) -> (path out=w540:path, error out=w545:errorcluster, "ImageBuf"=w544:u8[][][])  [unwired: 2 in, 2 out]
    n270 = flat-sequence {
      tunnel: [w608] -> w541
      frame #0 {
      }
      frame #1 {
        n271 = event shown="[1] \"停止\": 值改变" {
          selector: _ -> [_ _]
          dyn-events: _ -> [_ _]
          timeout: 0 -> [_ _]
          tunnel: [FALSE w611] -> w608
          event Timeout {
            n272 = event-data() -> ()  [unwired: 1 in, 2 out]
          }
          event "停止": Value Change {
            n273 = event-data() -> ("NewVal"=w612:bool)  [unwired: 1 in, 1 out]
            n274 = case shown="真" w612 {
              selector: w612 -> [_ w614]
              tunnel: [FALSE w614] -> w611
              frame False {
              }
              frame True {
                n275 = local write "开始/暂停"(w614) -> ()
                "停止循环" <- w614
              }
            }
          }
        }
      }
    }
    n276 = Index Array(array=w544) -> (element=w537:u8[][])  [unwired: 3 in]
    n277 = call "IMAQ ArrayToImage"("Image Pixels (U8)"=w537, "Image"=w542) -> ("Image Out"=w533:T1)  [unwired: 4 in, 5 out]
    "Image" <- w533
    n278 = Send Notification(notification=w537, notifier=w546, error in (no error)=w545) -> (error out=w543:errorcluster)  [unwired: 1 out]
    n279 = flat-sequence {
      tunnel: w533 -> [w574]
      tunnel: [w574] -> w532
      tunnel: [w583] -> w535
      tunnel: w532 -> [w584]
      tunnel: [w592] -> w534
      tunnel: w535 -> [w592]
      tunnel: w534 -> [w599]
      frame #0 {
        n280 = property on="Image" class="ImageControl"() -> ("Last Mouse Position"=w552:cluster{"X":i32, "Y":i32})  [unwired: 2 in, 2 out]
        n281 = call "IMAQ ImageToArray"("Optional Rectangle"=i32[] [647, 185, 658, 186], "Image"=w574) -> ("Image Pixels (U8)"=w570:u8[][])  [unwired: 2 in, 4 out]
        n282 = call "IMAQ ImageToArray"("Optional Rectangle"=i32[] [647, 425, 658, 426], "Image"=w574) -> ("Image Pixels (U8)"=w566:u8[][])  [unwired: 2 in, 4 out]
        n283 = for {
          tunnel: w570 -> [w579] mode=indexing
          shift-right: [w580] -> w564
          shift-left: u8[] [] -> [w578]
          n284 = Build Array (concatenate)(w578, w579) -> (w580:u8[])
        }
        n285 = for {
          tunnel: w566 -> [w576] mode=indexing
          shift-right: [w577] -> w565
          shift-left: u8[] [] -> [w575]
          n286 = Build Array (concatenate)(w575, w576) -> (w577:u8[])
        }
        n287 = Unbundle By Name(w552) -> ("X"=w573:i32, "Y"=w572:i32)
        n288 = call "IMAQ GetPixelValue"("Image"=w574, "X Coordinate"=w573, "Y Coordinate"=w572) -> ("Pixel Value (U8)"=w556:u8)  [unwired: 3 in, 4 out]
        n289 = call <vilib>:"Mean.vi"("X"=w564) -> ("mean"=w562:dbl)  [unwired: 1 out]
        n290 = call <vilib>:"Mean.vi"("X"=w565) -> ("mean"=w555:dbl)  [unwired: 1 out]
        n291 = Subtract(x="上限温度", y="下限温度") -> (x-y=w561:dbl)
        n292 = Subtract(x=w562, y=w555) -> (x-y=w560:dbl)
        n293 = Subtract(x=w556, y=w555) -> (x-y=w554:dbl)
        n294 = Divide(x=w561, y=w560) -> (x/y=w559:dbl)
        n295 = Multiply(x=w559, y=w554) -> (x*y=w558:dbl)
        n296 = Add(x="下限温度", y=w558) -> (x+y=→"当前点温度":dbl)
      }
      frame #1 {
        n297 = call "IMAQ Quantify 2"("Image Mask"="mask 1", "Image"=w584) -> ("Global Report"=w585:T7)  [unwired: 7 in, 2 out]
        n298 = call "IMAQ Quantify 2"("Image Mask"="mask 2", "Image"=w584) -> ("Global Report"=w586:T7)  [unwired: 7 in, 2 out]
        n299 = Unbundle By Name(w585) -> ("Mean Value"=w587:sgl)
        n300 = Unbundle By Name(w586) -> ("Mean Value"=w588:sgl)
        n301 = Subtract(x=w587, y=w588) -> (x-y=w589:sgl)
        n302 = In Range and Coerce(upper limit=sgl 5.0 ("上限"), x=w589, lower limit=sgl -5.0 ("下限")) -> (In Range?=w583:bool)  [unwired: 1 out]
      }
      frame #2 {
        n303 = local read "校准"() -> (w596:bool)
        n304 = Not Equal?(x=w592, y=w596) -> (x != y?=w595:bool)
        n305 = case shown="真" w595 {
          tunnel: [FALSE w598] -> w593
          tunnel: w592 -> [_ w598]
          frame False {
          }
          frame True {
          }
        }
        "start calibrate" <- w593
        n306 = call "已用时间"("Reset"=w593) -> ("Elapsed Time (s)"=→"校正循环计时":dbl)  [unwired: 4 in, 14 out]
      }
      frame #3 {
        "校准" <- w599
      }
    }
    n307 = call "Histogram.vi"("8-bit pixmap"=w537) -> ("Histogram Graph"=→"Histogram Graph":T2)  [unwired: 10 out]
    n308 = event shown="[1] \"Brightness\", \"Contrast\": 值改变" {
      selector: _ -> [_ _]
      dyn-events: _ -> [_ _]
      timeout: 0 -> [_ _]
      tunnel: w540 -> [w600 w607]
      tunnel: [w600 w606] -> w539
      event Timeout {
        n309 = event-data() -> ()  [unwired: 3 out]
      }
      event "Brightness", "Contrast": Value Change {
        n310 = event-data() -> ()  [unwired: 7 out]
        n311 = local read "Saturation"() -> (w605:i32)
        n312 = local read "Hue"() -> (w604:i32)
        n313 = dll-call lib="PTH1babs C\nProgram Files\tHikvision+DS-4000系列板卡SDK and Demo Version 5.1Bin\nDs40xxSDK.dll" fn="SetVideoPara"(path in=w607, "hChannelHandle"=u32 0, "Brightness"="Brightness", "Contrast"="Contrast", "Saturation"=w605, "Hue"=w604) -> (path out=w606:path)  [unwired: 7 in, 2 out]
      }
    }
  }
  n314 = dll-call lib="PTH1labs C\nProgram Files\tHikvision+DS-4000系列板卡SDK and Demo Version 5.1SDKcard sdk\nDs40xxSDK.dll" fn="DeInitDSPs"(path in=w4, error in=w5) -> (error out=→"错误输出":errorcluster, "返回类型"=→"DeInitDSPs":i32)  [unwired: 1 in, 1 out]
